vi "Data handler-Acquisition protocols.vi"(0 "Data-gen queue":T2, 2 "UI queue":refnum<queue>, 4 "Channel info":T1, 5 "Number of files closed in in":u32, 9 "Logging queue element in":T3={"Imaging Protocol"=enum."Live Imaging", "Number of Trials"=0, "Frame Size"=512, "# Averaged frames"=0, "Dwell time (us)"=0.0, "Index of Z-plane"=0, "Timelapse?"=FALSE, "Logging process is active"=FALSE, "Speed logging enabled"=FALSE, "tdms file ref"=refnum, "path"=path "", "Trial Number"=0, "Expected # points acquired"=FALSE, "Manually stopped"=FALSE, "Ch0 data"=[], "Ch1 data"=[], "Last trial"=FALSE, "Points acquired"={"Ch0 last trial"=0, "Ch1 last trial"=0, "All trials"=0}} {"Frame Size" items=["100X100"=100, "128X128"=128, "200X200"=200, "256X256"=256, "512X512"=512, "1024x1024"=1024, "2048x2048"=2048]; "Dwell time (us)" format="%#.6g"}) -> (6 "Number of files closed out":u32, 15 "error out":errorcluster)   [LabVIEW 2013]
uses:
  Typedefs/Logging queue element.ctl
  Typedefs/Imaging Protocols enum.ctl
  Typedefs/Frame Size.ctl
  Typedefs/Acquired points count.ctl
  Typedefs/ROI File Generator Queue Ref.ctl
  User Interface/Queue/Message Queue/Typedefs/Message Cluster.ctl
panel:
  out "Last trial?":bool
  out "Expected # points acquired":bool
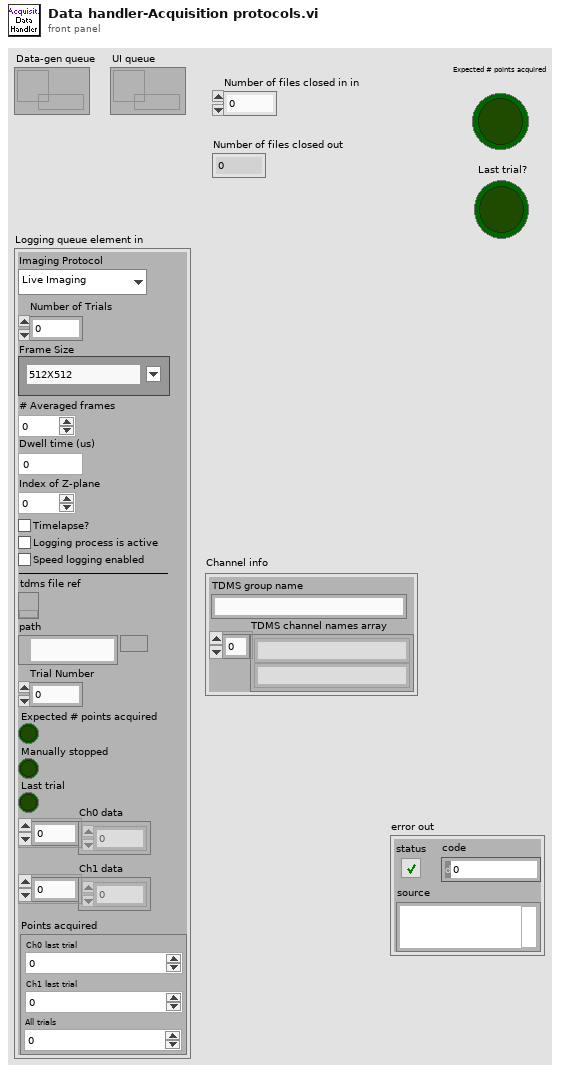
[diagram p1: front panel]
types:
  T1 = cluster{"TDMS group name":string, "TDMS channel names array":string[]}
  T2 = typedef "ROI File Generator Queue Ref.ctl" = refnum<queue>
  T3 = typedef "Logging queue element.ctl" = cluster{"Imaging Protocol":T4, "Number of Trials":u16, "Frame Size":T5, "# Averaged frames":u16, "Dwell time (us)":dbl, "Index of Z-plane":i32, "Timelapse?":bool, "Logging process is active":bool, "Speed logging enabled":bool, "tdms file ref":refnum<k34>, "path":path, "Trial Number":i32, "Expected # points acquired":bool, "Manually stopped":bool, "Ch0 data":u32[], "Ch1 data":u32[], "Last trial":bool, "Points acquired":T6}
  T4 = typedef "Imaging Protocols enum.ctl" = enum16{"AOL Z-Stack", "Motor Z Stack", "Functional Acquisition", "Single Plane Acquisition", "Volume Acquisition", "Live Imaging", "Live Plane Imaging", "Live Volume Imaging"}
  T5 = typedef "Frame Size.ctl" = u16
  T6 = typedef "Acquired points count.ctl" = cluster{"Ch0 last trial":u64, "Ch1 last trial":u64, "All trials":u64}
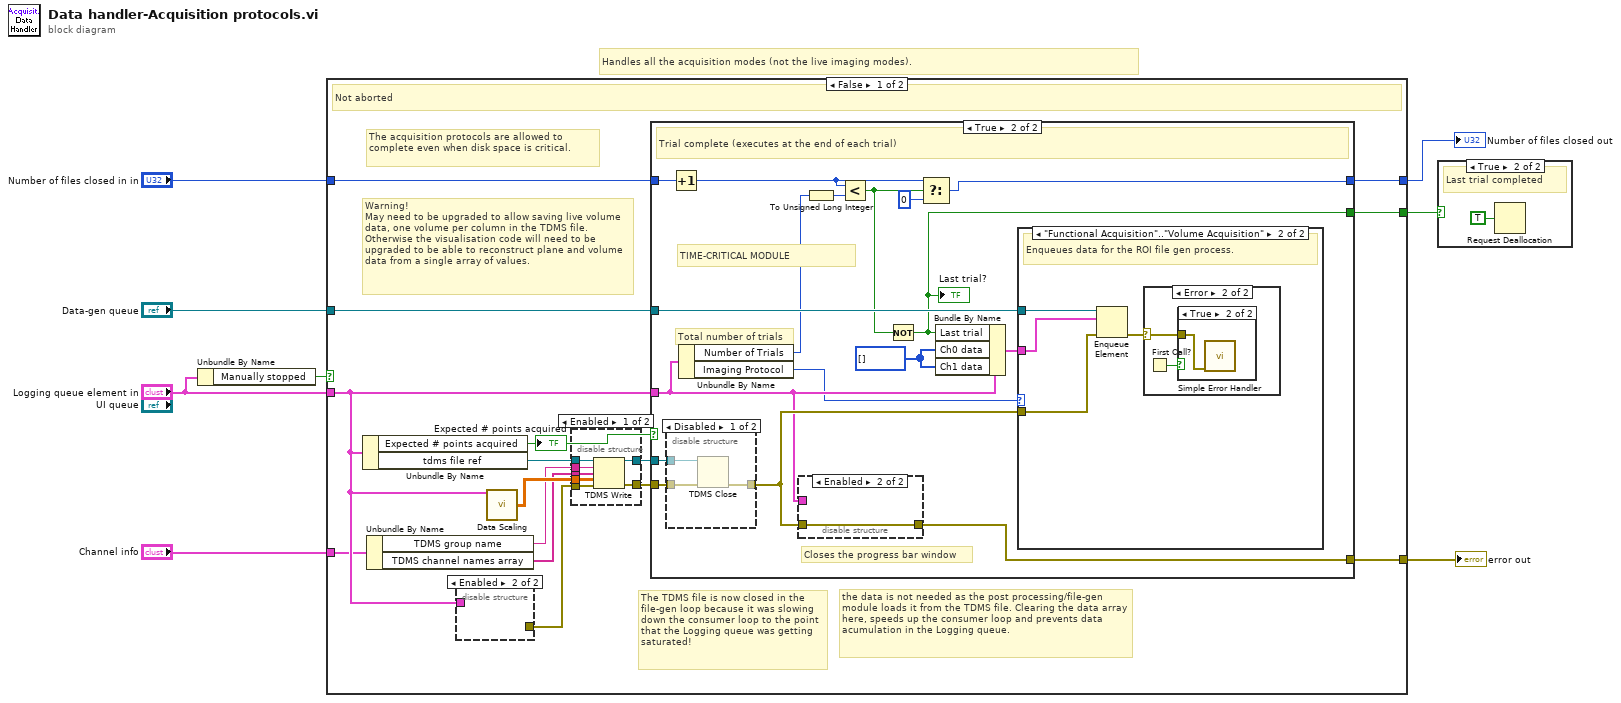
[diagram p0: block diagram]
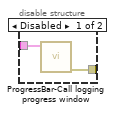
[diagram p3: hidden frame]
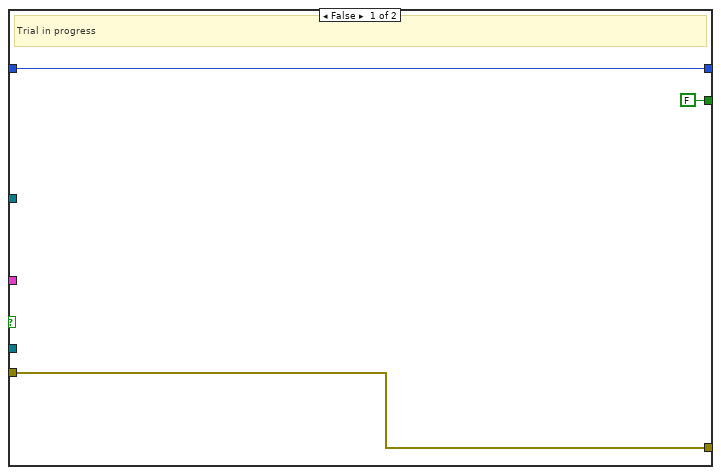
[diagram p4: hidden frame]
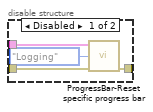
[diagram p8: hidden frame]
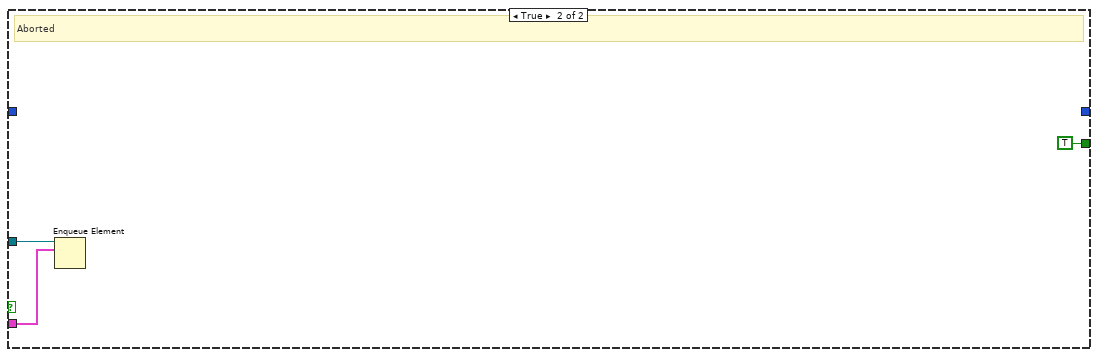
[diagram p10: hidden frame]
diagram:
  # "Handles all the acquisition modes (not the live imaging modes)."
  n1 = Unbundle By Name("Logging queue element in") -> ("Manually stopped"=w2:bool)
  n2 = case shown="False" w2 {
    tunnel: "Data-gen queue" -> [w23 w70]
    tunnel: [w22 _] -> w7
    tunnel: "Number of files closed in in" -> [w21 _]
    tunnel: "Logging queue element in" -> [w15 w69]
    tunnel: [w14 _] -> w1
    tunnel: [w13 TRUE] -> w5
    tunnel: "Channel info" -> [w11 _]
    frame False {
      # "The TDMS file is now closed in the file-gen loop because it was slowing down the consumer loop to the point that the Logging queue was getting saturated!"
      # "the data is not needed as the post processing/file-gen module loads it from the TDMS file. Clearing the data array here, speeds up the consumer loop and prevents data acumulation in the Logging queue."
      # "The acquisition protocols are allowed to complete even when disk space is critical."
      # "Warning!\nMay need to be upgraded to allow saving live volume data, one volume per column in the TDMS file. Otherwise the visualisation code will need to be upgraded to be able to reconstruct plane and volume data from a single array of values."
      # "Not aborted"
      n3 = Unbundle By Name(w15) -> ("Expected # points acquired"=w17:bool, "tdms file ref"=w18:refnum<k34>)
      "Expected # points acquired" <- w17
      n4 = Unbundle By Name(w11) -> ("TDMS group name"=w10:string, "TDMS channel names array"=w9:string[])
      n5 = disable-structure shown="Enabled" {
        disable-tunnel: [w32 _] -> w16
        disable-tunnel: w15 -> [w31 _]
        frame Disabled {
          n6 = call "ProgressBar-Call logging progress window.vi"("Z-stack queue cluster"=w31) -> ("error out"=w32:errorcluster)  [unwired: 10 in]
        }
        frame Enabled {
        }
      }
      n7 = call "Data Scaling.vi"("Logging queue element in"=w15) -> ("Two channel data"=w12:dbl[][])  [unwired: 13 in, 1 out]
      n8 = disable-structure shown="Enabled" {
        disable-tunnel: [w30 _] -> w20
        disable-tunnel: [w29 _] -> w19
        disable-tunnel: w18 -> [w28 _]
        disable-tunnel: w9 -> [w27 _]
        disable-tunnel: w10 -> [w26 _]
        disable-tunnel: w16 -> [w25 _]
        disable-tunnel: w12 -> [w24 _]
        frame Enabled {
          n9 = TDMS Write(0:w28, 5:w26, 7:w27, 9:w24, 11:w25) -> (4:w29:refnum<k34>, 15:w30:errorcluster)  [unwired: 1 in, 2 out]
        }
        frame Disabled {
        }
      }
      n10 = case shown="True" w17 {
        tunnel: w20 -> [w35 w52]
        tunnel: w19 -> [_ w51]
        tunnel: [w35 w36] -> w14
        tunnel: w23 -> [_ w50]
        tunnel: w15 -> [_ w42]
        tunnel: [w34 w46] -> w22
        tunnel: w21 -> [w34 w49]
        tunnel: [FALSE w39] -> w13
        frame False {
          # "Trial in progress"
        }
        frame True {
          w37 = u32[] [] ("Raw Data")
          # "TIME-CRITICAL MODULE"
          # "Total number of trials"
          # "Closes the progress bar window"
          # "Trial complete (executes at the end of each trial)"
          n11 = disable-structure shown="Disabled" {
            disable-tunnel: w52 -> [w67 w68]
            disable-tunnel: w51 -> [w66 _]
            disable-tunnel: [w65 w68] -> w48
            frame Disabled {
              n12 = TDMS Close(8:w67, 11:w66) -> (0:w65:errorcluster)  [unwired: 1 out]
            }
            frame Enabled {
            }
          }
          n13 = Increment(x=w49) -> (x+1=w40:u32)
          n14 = Unbundle By Name(w42) -> ("Number of Trials"=w47:u16, "Imaging Protocol"=w38:T4)
          n15 = disable-structure shown="Enabled" {
            disable-tunnel: [w62 w64] -> w36
            disable-tunnel: w48 -> [w61 w64]
            disable-tunnel: w42 -> [w60 _]
            frame Disabled {
              n16 = call "ProgressBar-Reset specific progress bar.vi"("Error in"=w61, "Sender"=enum16{"Acquisition", "Logging", "File gen"}."Logging", "Z-stack queue cluster"=w60) -> ("error out"=w62:errorcluster)  [unwired: 8 in]
            }
            frame Enabled {
            }
          }
          n17 = To Unsigned Long Integer(number=w47) -> (unsigned 32bit integer=w44:u32)
          n18 = Less?(x=w40, y=w44) -> (x < y?=w43:bool)
          n19 = Not(x=w43) -> (.not. x?=w39:bool)
          "Last trial?" <- w39
          n20 = Select(t=w40, s=w43, f=u32 0) -> (s? t:f=w46:u32)
          n21 = Bundle By Name(cluster=w42, "Last trial"=w39, "Ch0 data"=w37, "Ch1 data"=w37) -> (w41:T3)
          n22 = case shown="\"Functional Acquisition\"..\"Volume Acquisition\"" w38 {
            tunnel: w48 -> [_ w54]
            tunnel: w50 -> [_ w56]
            tunnel: w41 -> [_ w53]
            frame Default {
              # "Unhandled modes"
            }
            frame "Functional Acquisition".."Volume Acquisition" {
              # "Enqueues data for the ROI file gen process."
              n23 = Enqueue Element(queue=w56, element=w53, error in (no error)=w54) -> (error out=w55:errorcluster)  [unwired: 1 in, 2 out]
              n24 = case shown="Error" w55 {
                selector: w55 -> [_ w58]
                frame No Error {
                }
                frame Error {
                  n25 = First Call?() -> (First Call?: T/F=w57:bool)
                  n26 = case shown="True" w57 {
                    tunnel: w58 -> [_ w59]
                    frame False {
                    }
                    frame True {
                      n27 = call <vilib>:"Simple Error Handler.vi"("error in (no error)"=w59) -> ()  [unwired: 4 in, 5 out]
                    }
                  }
                }
              }
            }
          }
        }
      }
    }
    frame True {
      # "Aborted"
      n28 = Enqueue Element(queue=w70, element=w69) -> ()  [unwired: 2 in, 3 out]
    }
  }
  "error out" <- w1
  "Number of files closed out" <- w7
  n29 = case shown="True" w5 {
    frame False {
    }
    frame True {
      # "Last trial completed"
      n30 = Request Deallocation(TRUE ("flag")) -> ()
    }
  }
